vi "Add Result Channels.vi"(8 "error in (no error)":errorcluster, 9 "Selected Source Waveform items":T1[](array[typedef]) format="%.0x", 10 "Selected Waveform Result Section Items":T1[](array[typedef]) format="%.0x", 11 "ScaledWaveformCalculation in":refnum<class "ScaledWaveformCalculation.lvclass">) -> (0 "error out":errorcluster, 3 "ScaledWaveformCalculation out":refnum<class "ScaledWaveformCalculation.lvclass">)   [LabVIEW 2015, in "ScaledWaveformCalculation.lvclass"]
uses:
  Waveform-Processing-Custom-Device Configuration.llb/ScaledWaveformCalculation.lvclass
  Waveform-Processing-Custom-Device Configuration.llb/Custom Device Item Ref.ctl
  Waveform-Processing-Custom-Device Configuration.llb/WaveformCalculation.lvclass/WaveformCalculation.ctl
  Waveform-Processing-Custom-Device Configuration.llb/Custom Device Waveform.ctl
  Waveform-Processing-Custom-Device Configuration.llb/Custom Device Waveform DataType.ctl
  Waveform-Processing-Custom-Device Configuration.llb/WaveformCalculation.lvclass
  Waveform-Processing-Custom-Device Configuration.llb/Custom Device API.lvlib
  Waveform-Processing-Custom-Device Configuration.llb/Waveform-Processing-Custom-Device System Explorer.lvlib
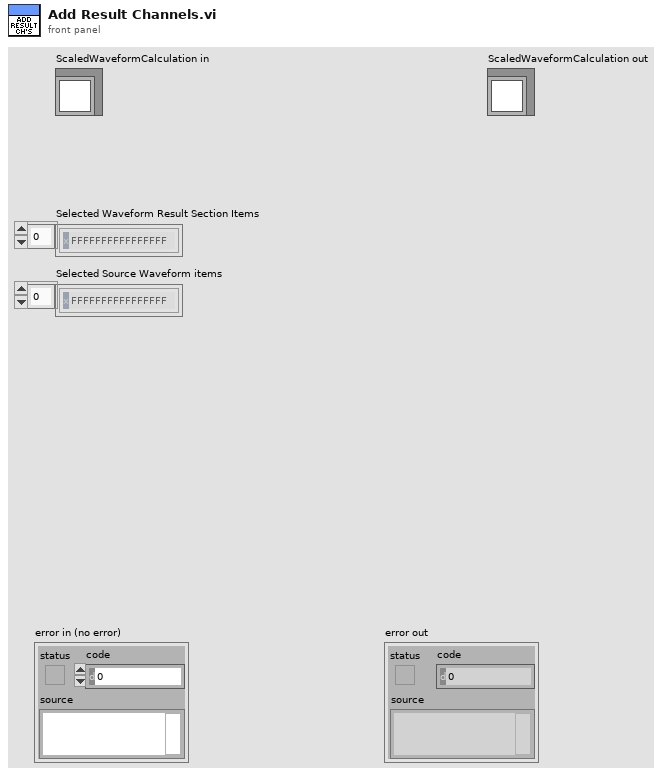
[diagram p1: front panel]
types:
  T1 = typedef "Custom Device API.lvlib/Custom Device Item Ref.ctl" = u64
  T2 = typedef "Custom Device API.lvlib/Custom Device Waveform.ctl" = cluster{"Data Type":T3, "Units":string}
  T3 = typedef "Custom Device API.lvlib/Custom Device Waveform DataType.ctl" = enum16{"Double", "Complex Double"}
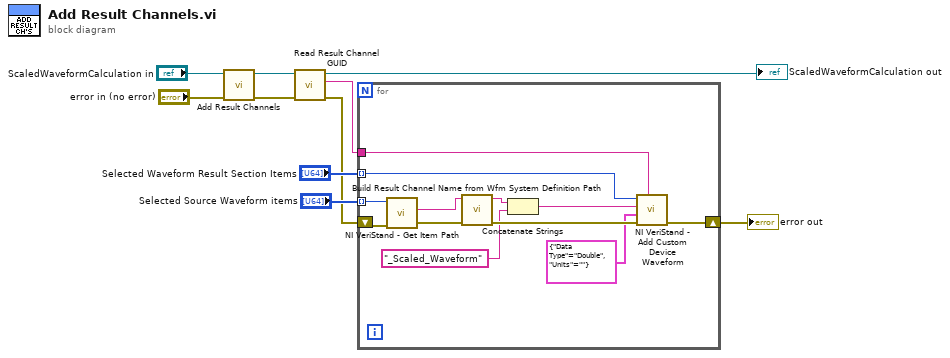
[diagram p0: block diagram]
diagram:
  n1 = call-parent "Add Result Channels.vi"("error in (no error)"="error in (no error)", "WaveformCalculation in"="ScaledWaveformCalculation in") -> ("error out"=w8:errorcluster, "WaveformCalculation out"=w7:refnum<class "ScaledWaveformCalculation.lvclass">)  [unwired: 8 in]
  n2 = call "Read Result Channel GUID.vi"("error in (no error)"=w8, "WaveformCalculation in"=w7) -> ("error out"=w4:errorcluster, "Result Channel GUID"=w1:string, "WaveformCalculation out"=→"ScaledWaveformCalculation out":refnum<class "ScaledWaveformCalculation.lvclass">)  [unwired: 7 in]
  n3 = for {
    tunnel: "Selected Source Waveform items" -> [w21] mode=indexing
    tunnel: "Selected Waveform Result Section Items" -> [w17] mode=indexing
    shift-right: [w15] -> w3
    shift-left: w4 -> [w22]
    tunnel: w1 -> [w11]
    n4 = call "NI VeriStand - Get Item Path.vi"("error in (no error)"=w22, "Item Ref in"=w21) -> ("error out"=w20:errorcluster, "Path"=w19:string)  [unwired: 6 in, 2 out]
    n5 = call "Build Result Channel Name from Wfm System Definition Path.vi"("error in (no error)"=w20, "Channel Path"=w19) -> ("error out"=w18:errorcluster, "delimited string"=w13:string)  [unwired: 8 in]
    n6 = Concatenate Strings(w13, "_Scaled_Waveform" ("string")) -> (w12:string)
    n7 = call "NI VeriStand - Add Custom Device Waveform.vi"("GUID (Default Waveform)"=w11, "error in (no error)"=w18, "Waveform"=T2 {"Data Type"=enum."Double", "Units"=""}, "Waveform Name"=w12, "Parent Ref in"=w17) -> ("error out"=w15:errorcluster)  [unwired: 3 in, 3 out]
  }
  "error out" <- w3
